vi "writeVar.vi"(8 "错误输入（无错误）":errorcluster, 9 "var":string, 10 "id":u16, 11 "TCP网络连接输入":refnum<k5>) -> (0 "错误输出":errorcluster, 1 "data out":string, 3 "TCP网络连接输出":refnum<k5>)   [LabVIEW 2015, in "labOpenShowVar.lvlib"]
uses:
  labOpenShowVar.lvlib
panel:
  in  "val":string
  out "baseData":u8[](array[numeric])
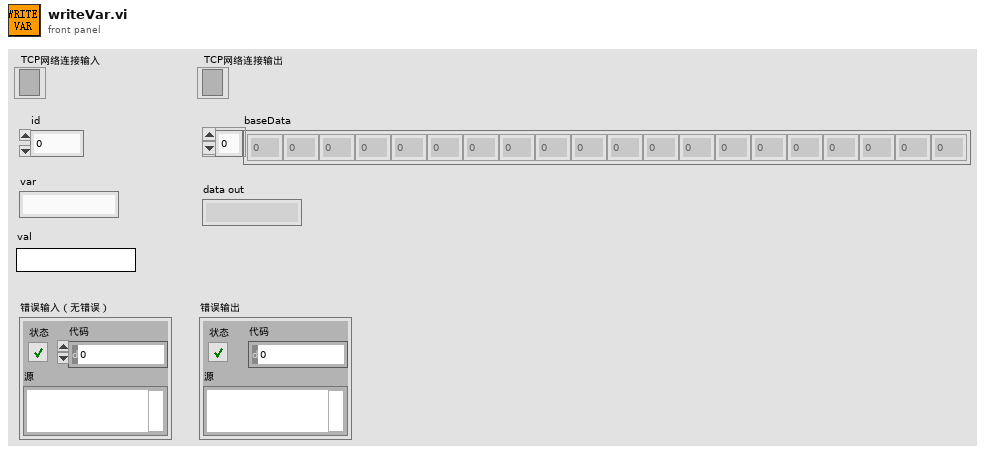
[diagram p1: front panel]
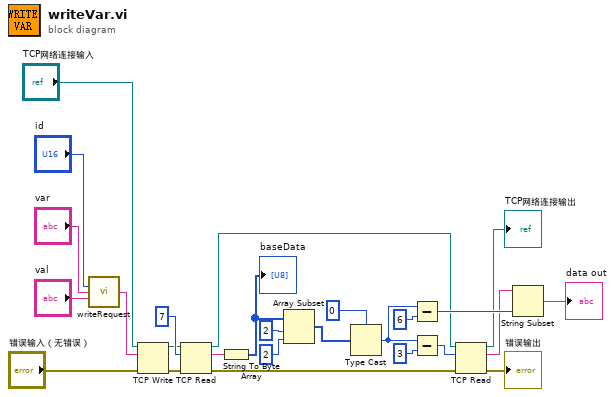
[diagram p0: block diagram]
diagram:
  n1 = call "writeRequest.vi"("id"="id", "cmd"="var", "data"="val") -> ("readRequest"=w5:string)  [unwired: 12 in]
  n2 = TCP Write(connection ID="TCP网络连接输入", data in=w5, error in (no error)="错误输入（无错误）") -> (connection ID out=w7:refnum<k5>, error out=w8:errorcluster)  [unwired: 1 in, 1 out]
  n3 = TCP Read(connection ID=w7, bytes to read=7 ("读取的字节"), error in (no error)=w8) -> (connection ID out=w15:refnum<k5>, data out=w10:string, error out=w16:errorcluster)  [unwired: 2 in]
  n4 = String To Byte Array(string=w10) -> (unsigned byte array=w19:u8[])
  "baseData" <- w19
  n5 = Array Subset(array=w19, index=2 ("索引"), length=2 ("长度")) -> (w13:u8[])
  n6 = Type Cast(type=i16 0, x=w13) -> (*(type *) &x=w24:i16)
  n7 = Subtract(x=w24, y=i16 6) -> (x-y=w22:i16)
  n8 = Subtract(x=w24, y=i16 3) -> (x-y=w20:i16)
  n9 = TCP Read(connection ID=w15, bytes to read=w20, error in (no error)=w16) -> (connection ID out=→"TCP网络连接输出":refnum<k5>, data out=w21:string, error out=→"错误输出":errorcluster)  [unwired: 2 in]
  n10 = String Subset(string=w21, length (rest)=w22) -> (substring=→"data out":string)  [unwired: 1 in]
